vi "pakistan.vi"() -> ()   [LabVIEW 2011]
uses:
  <vilib>/imath/engines/lvmath2/RunTimeEngine/ErrorHandling/NIMS_Finalize Error.vi
  <vilib>/imath/engines/lvmath2/RunTimeEngine/Managers/WorkSpace/UID Generator.vi
  <vilib>/imath/engines/lvmath2/RunTimeEngine/Managers/SymbolTable/Clear UID.vi
  <vilib>/imath/engines/lvmath2/RunTimeEngine/NodeEndStatement/NIMS_NodeEndStatement_Output.vi
  <instcachedir>/0/NIMS_NodeEndStatement_Output_53EC0D466D134D7ABD903AC30B43404B.lvgen/NIMS_NodeEndStatement_Output_53EC0D466D134D7ABD903AC30B43404B_001.vi
  <vilib>/imath/engines/lvmath2/RunTimeEngine/RunTimeType/NIMS_RunTimeType_From StrictType (excl LVString).vi
  <instcachedir>/0/NIMS_RunTimeType_From StrictType (excl LVString)_46AE8B54A11948F0BCCEB8091EE7AA4C.lvgen/NIMS_RunTimeType_From StrictType (excl LVString)_46AE8B54A11948F0BCCEB8091EE7AA4C_000.vi
  <vilib>/imath/engines/lvmath2/RunTimeEngine/LocalVariableDefStatement/MC_LocalVariableDefStatement_Display.vi
  GloryofPakistan/VisualStudio/linking/Debug/linking.dll
  <vilib>/imath/engines/lvmath2/RunTimeEngine/Managers/SymbolTable/NIMS_WorkSpace.lvlib
panel:
  out "Soup":dbl
  in  "Carrots":dbl
  in  "Water":dbl
  in  "Boolean 2":bool
  out "X^2 + Y^2":dbl
  in  "X":dbl
  in  "Y":dbl
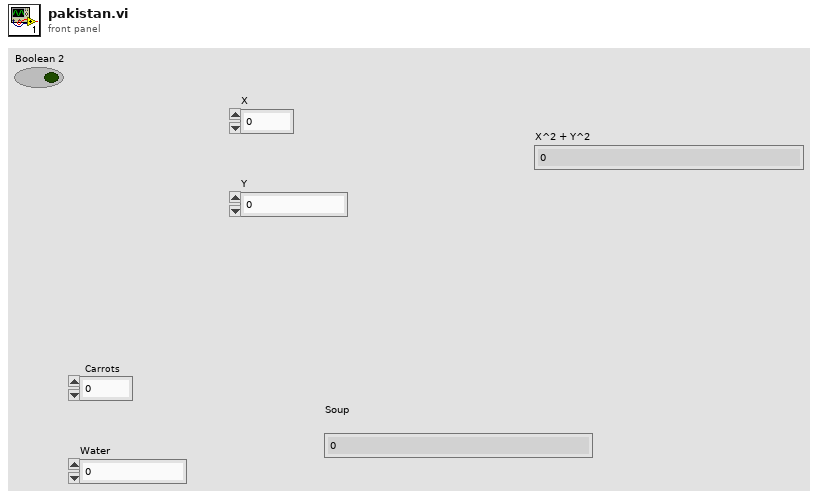
[diagram p1: front panel]
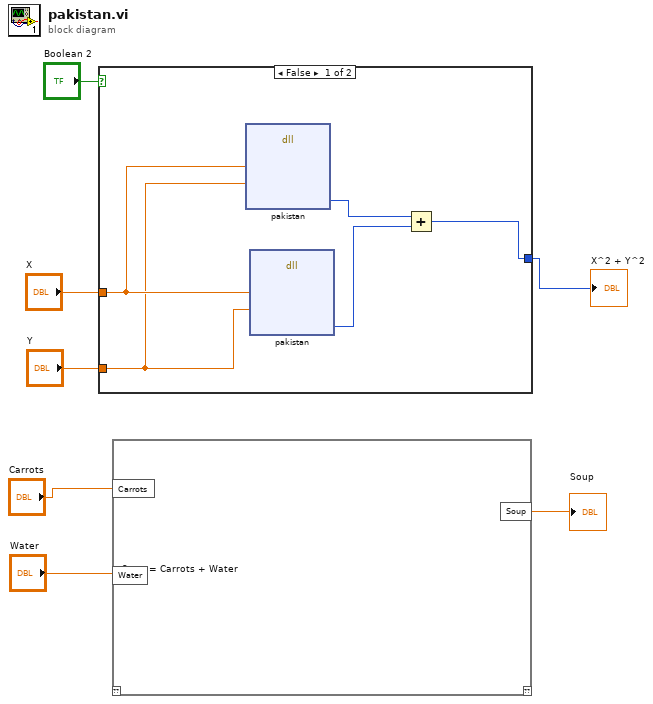
[diagram p0: block diagram]
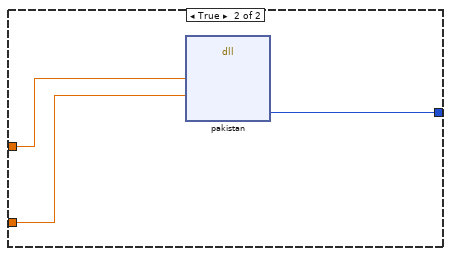
[diagram p2: hidden frame]
diagram:
  n1 = case shown="False" "Boolean 2" {
    tunnel: "X" -> [w10 w15]
    tunnel: "Y" -> [w9 w14]
    tunnel: [w8 w13] -> w5
    frame False {
      n2 = dll-call lib="C:/Users/umfehr44.ENG/Desktop/Micromirror Project/GloryofPakistan/VisualStudio/linking/Debug/linking.dll" fn="pakistan" ("False Fuction")("x"=w10, "y"=w9) -> ("z"=w12:i32)  [unwired: 7 in, 2 out]
      n3 = dll-call lib="C:/Users/umfehr44.ENG/Desktop/Micromirror Project/GloryofPakistan/VisualStudio/linking/Debug/linking.dll" fn="pakistan" ("False Fuction")("x"=w10, "y"=w9) -> ("z"=w11:i32)  [unwired: 7 in, 2 out]
      n4 = Add(x=w12, y=w11) -> (x+y=w8:i32)
    }
    frame True {
      n5 = dll-call lib="C:/Users/umfehr44.ENG/Desktop/Micromirror Project/GloryofPakistan/VisualStudio/linking/Debug/linking.dll" fn="pakistan"("x"=w15, "y"=w14) -> ("z"=w13:i32)  [unwired: 7 in, 2 out]
    }
  }
  "X^2 + Y^2" <- w5
  n6 = mathscript code="Soup = Carrots + Water"("Carrots"="Carrots", "Water"="Water") -> ("Soup"=→"Soup":dbl)  [unwired: 1 in, 1 out]
